vi "max30100_deneme3.vi"() -> ()   [LabVIEW 2017]
uses:
  <vilib>/Instr/_visa.llb/VISA Configure Serial Port (Instr).vi
panel:
  in  "Boolean 2":bool
  in  "Boolean":bool
  in  "stop":bool
  in  "VISA resource name":refnum<visa-resource-name>
  out "Numeric":dbl
  in  "OK Button":bool
  out "Waveform Chart":dbl(graph)
  out "Thermometer":dbl(slide) scale=0.0..100.0
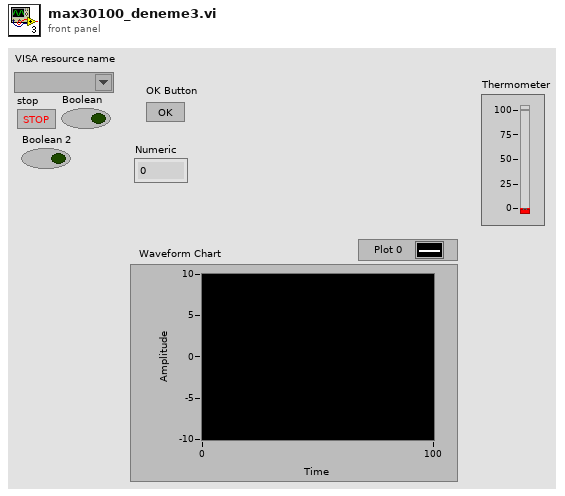
[diagram p1: front panel]
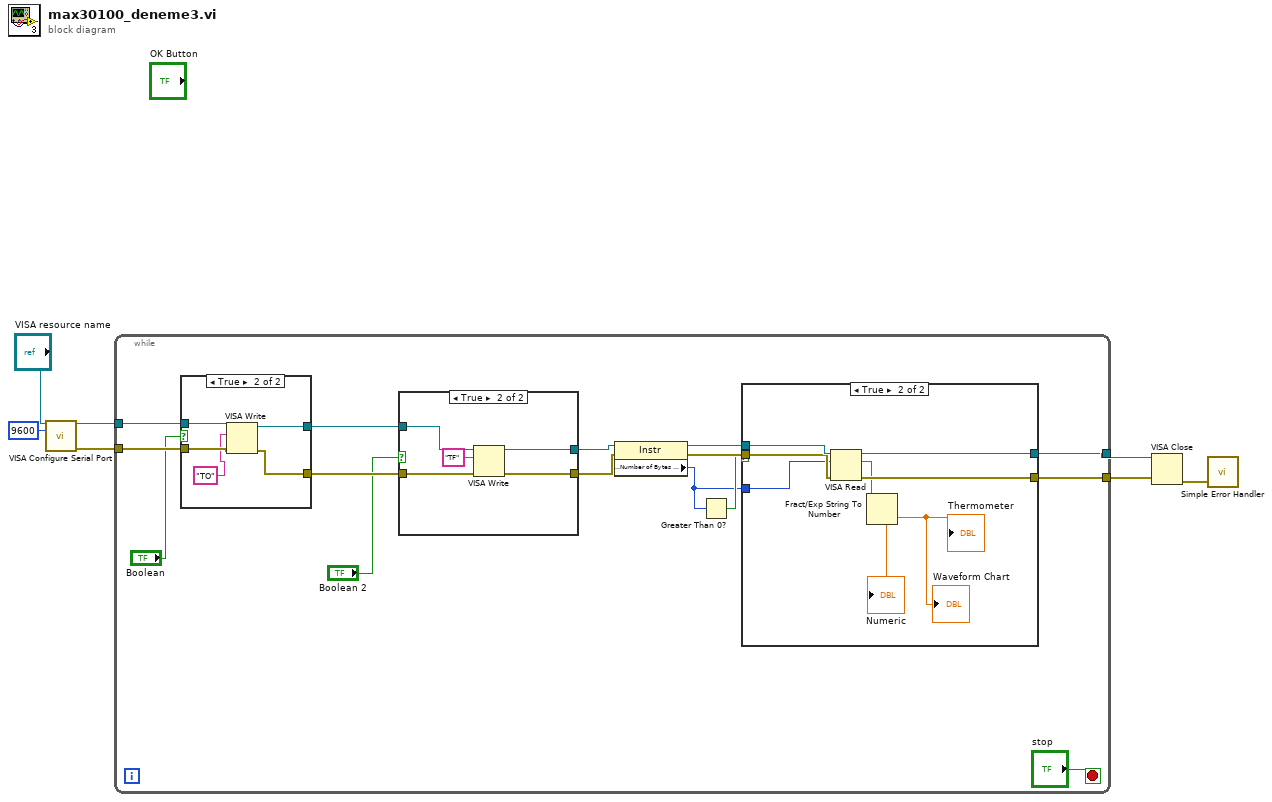
[diagram p0: block diagram]
diagram:
  n1 = call-poly "VISA Configure Serial Port"("VISA resource name"="VISA resource name", "baud rate (9600)"=u32 9600) -> ("VISA resource name out"=w7:refnum<visa-resource-name>, "error out"=w6:errorcluster)  [unwired: 12 in]
  n2 = while {
    tunnel: w7 -> [w20]
    tunnel: w6 -> [w19]
    tunnel: [w18] -> w5
    tunnel: [w17] -> w4
    stop <- "stop" stop-if-true
    n3 = case shown="True" "Boolean" {
      tunnel: [_ w39] -> w22
      tunnel: [_ w38] -> w21
      tunnel: w20 -> [_ w36]
      tunnel: w19 -> [_ w37]
      frame False {
      }
      frame True {
        n4 = VISA Write(VISA resource name=w36, write buffer="TO", error in (no error)=w37) -> (VISA resource name out=w39:refnum<visa-resource-name>, error out=w38:errorcluster)  [unwired: 1 out]
      }
    }
    n5 = case shown="True" "Boolean 2" {
      tunnel: w22 -> [_ w34]
      tunnel: w21 -> [_ w33]
      tunnel: [_ w32] -> w16
      tunnel: [_ w31] -> w15
      frame False {
      }
      frame True {
        n6 = VISA Write(VISA resource name=w34, write buffer="TF", error in (no error)=w33) -> (VISA resource name out=w32:refnum<visa-resource-name>, error out=w31:errorcluster)  [unwired: 1 out]
      }
    }
    n7 = property class="Instr"(reference=w16, error in=w15) -> (reference out=w14:refnum<visa-resource-name>, error out=w13:errorcluster, "Serial Settings:Number of Bytes at Serial Port"=w11:u32)
    n8 = Greater Than 0?(x=w11) -> (x > 0?=w12:bool)
    n9 = case shown="True" w12 {
      tunnel: [_ w29] -> w18
      tunnel: [_ w28] -> w17
      tunnel: w14 -> [_ w27]
      tunnel: w13 -> [_ w26]
      tunnel: w11 -> [_ w25]
      frame False {
      }
      frame True {
        n10 = VISA Read(VISA resource name=w27, byte count=w25, error in (no error)=w26) -> (VISA resource name out=w29:refnum<visa-resource-name>, read buffer=w24:string, error out=w28:errorcluster)  [unwired: 1 out]
        n11 = Fract/Exp String To Number(string=w24) -> (number=→"Thermometer" →"Waveform Chart" →"Numeric":dbl)  [unwired: 3 in, 1 out]
      }
    }
  }
  n12 = VISA Close(VISA resource name=w5, error in (no error)=w4) -> (error out=w1:errorcluster)
  n13 = call <vilib>:"Simple Error Handler.vi"("error in (no error)"=w1) -> ()  [unwired: 4 in, 5 out]
